vi "Memory.Array.Subset.vi"(7 "length (-1: rest)":i64 format="%d bytes", 8 "error in (no error)":errorcluster, 9 "index (0)":u64, 11 "Array in":refnum<class "Memory.Array.Void.lvclass">) -> (0 "error out":errorcluster, 2 "subset Array":refnum<class "Memory.Array.Void.lvclass">, 3 "Array out":refnum<class "Memory.Array.Void.lvclass">)   [LabVIEW 2016, in "Memory.Array.Void.lvclass"]
uses:
  Memory.Array.Void.lvclass
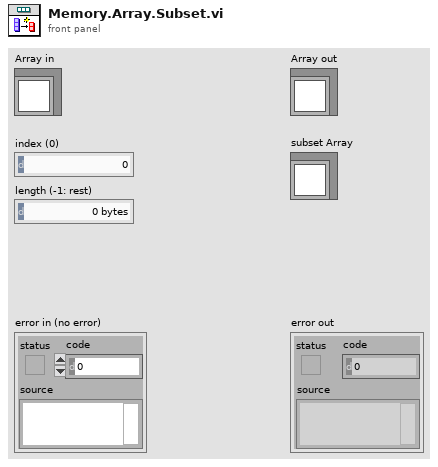
[diagram p1: front panel]
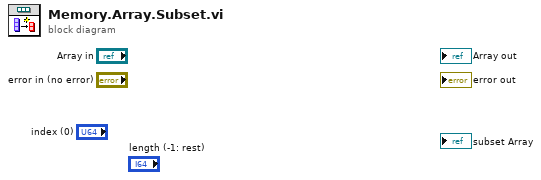
[diagram p0: block diagram]
diagram:
